vi "题目3.vi"(2 "停止":bool, 3 "温度单位":bool) -> (0 "温度":string, 1 "温度计":dbl(slide) scale=0.0..300.0)   [LabVIEW 2017]
panel:
  # "℉"
  # "℃"
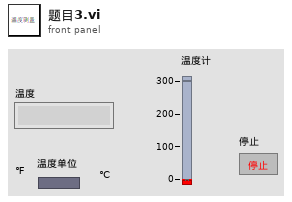
[diagram p1: front panel]
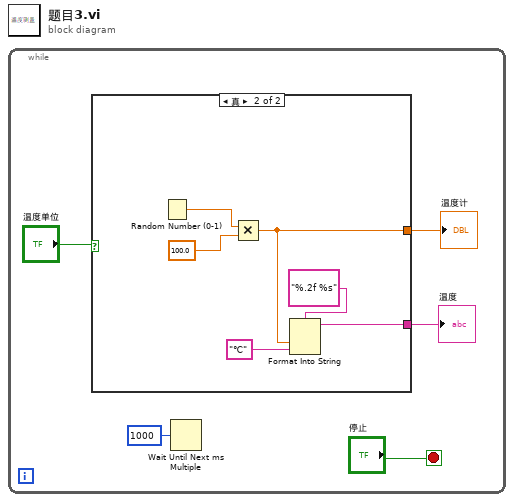
[diagram p0: block diagram]
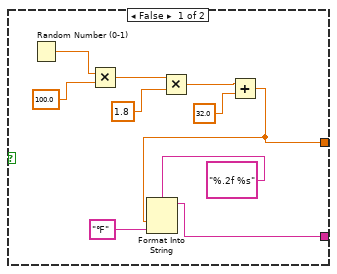
[diagram p2: hidden frame]
diagram:
  n1 = while {
    stop <- "停止" stop-if-true
    n2 = case shown="真" "温度单位" {
      tunnel: [w7 w19] -> w5
      tunnel: [w6 w16] -> w4
      frame False {
        n3 = Random Number (0-1)() -> (number: 0 to 1=w15:dbl)
        n4 = Multiply(x=w15, y=100.0) -> (x*y=w13:dbl)
        n5 = Multiply(x=w13, y=1.8) -> (x*y=w11:dbl)
        n6 = Add(x=w11, y=32.0) -> (x+y=w7:dbl)
        n7 = Format Into String(format string="%.2f %s", w7, "℉") -> (resulting string=w6:string)  [unwired: 2 in, 1 out]
      }
      frame True {
        n8 = Random Number (0-1)() -> (number: 0 to 1=w21:dbl)
        n9 = Multiply(x=w21, y=100.0) -> (x*y=w19:dbl)
        n10 = Format Into String(format string="%.2f %s", w19, "℃") -> (resulting string=w16:string)  [unwired: 2 in, 1 out]
      }
    }
    "温度计" <- w5
    "温度" <- w4
    n11 = Wait Until Next ms Multiple(millisecond multiple=u32 1000 ("毫秒倍数")) -> ()  [unwired: 1 out]
  }
